vi "Destroy Manager Subpanel.vi"(8 "error in (no error)":errorcluster, 11 "CIF_Manager_UI in":refnum<class "CIF_Manager_UI.lvclass">) -> (0 "error out":errorcluster, 3 "CIF_Manager_UI out":refnum<class "CIF_Manager_UI.lvclass">)   [LabVIEW 2021, in "CIF_Manager_UI.lvclass"]
uses:
  CIF_Manager_UI.lvclass
  CIF_Manager_UI.lvclass/CIF_Manager_UI.ctl
  <vilib>/CIF Foundation/CIF Core/CIFUI/CIF_UI.lvclass
  C:/Program Files/National Instruments/LabVIEW 2021/vi.lib/CIF Foundation/CIF Core/CIFUI/CIF_UI.lvclass
  D:/dev/CIF_Manager/src/CIFPluginManager/UI/CIFManagerUI Class/CIF_Manager_UI.lvclass
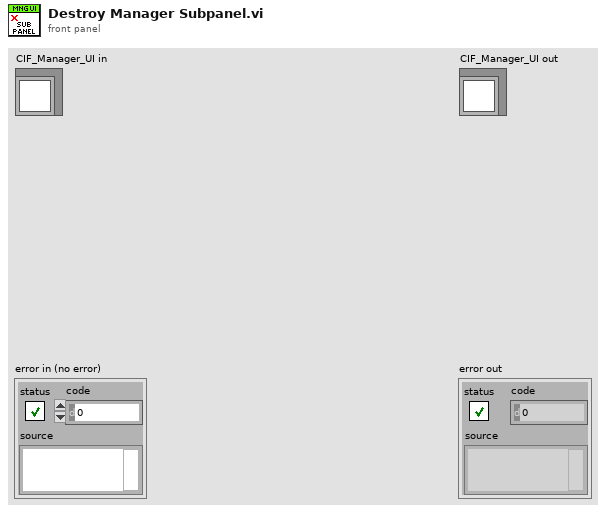
[diagram p1: front panel]
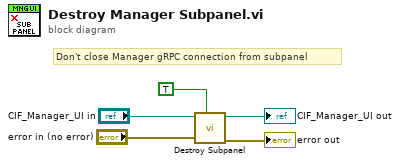
[diagram p0: block diagram]
diagram:
  # "Don't close Manager gRPC connection from subpanel"
  n1 = call <vilib>:"Destroy Subpanel.vi"("Skip Manager Close"=TRUE, "error in (no error)"="error in (no error)", "CIF_UI in"="CIF_Manager_UI in") -> ("error out"=→"error out":errorcluster, "CIF_UI out"=→"CIF_Manager_UI out":refnum<class "CIF_Manager_UI.lvclass">)  [unwired: 7 in]
